vi "Windspeed Warnings.vi"(8 "error in":errorcluster, 11 "Weather Data In":T1={"Current Temperature"=0.0, "Max Temperature"=0.0, "Min Temperature"=0.0, "Temperature Warning?"=FALSE, "Temperature Warning Text"="No Warning", "Current Windspeed"=0.0, "Max Windspeed"=0.0, "Windspeed Warning?"=FALSE, "Windspeed Warning Text"="No Warning"}) -> (0 "error out":errorcluster, 3 "Weather Data Out":T1={"Current Temperature"=0.0, "Max Temperature"=0.0, "Min Temperature"=0.0, "Temperature Warning?"=FALSE, "Temperature Warning Text"="No Warning", "Current Windspeed"=0.0, "Max Windspeed"=0.0, "Windspeed Warning?"=FALSE, "Windspeed Warning Text"="No Warning"})   [LabVIEW 2012]
doc: "This VI is used to determine the string to output to the weather station based on the current wind and limit settings."
uses:
  Weather Data.ctl
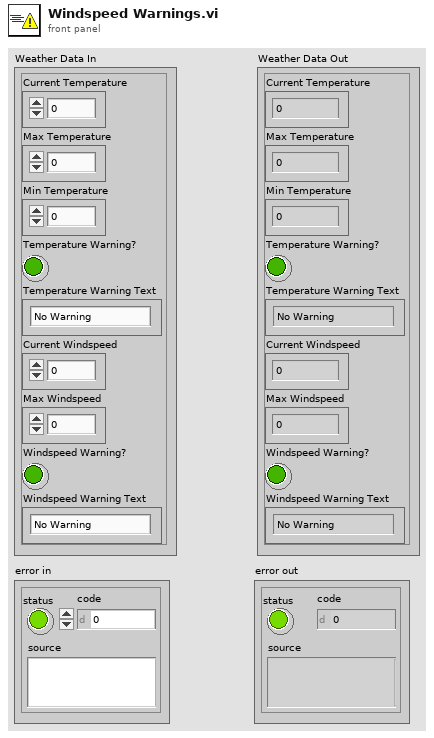
[diagram p1: front panel]
types:
  T1 = typedef "Weather Data.ctl" = cluster{"Current Temperature":dbl, "Max Temperature":dbl, "Min Temperature":dbl, "Temperature Warning?":bool, "Temperature Warning Text":string, "Current Windspeed":dbl, "Max Windspeed":dbl, "Windspeed Warning?":bool, "Windspeed Warning Text":string}
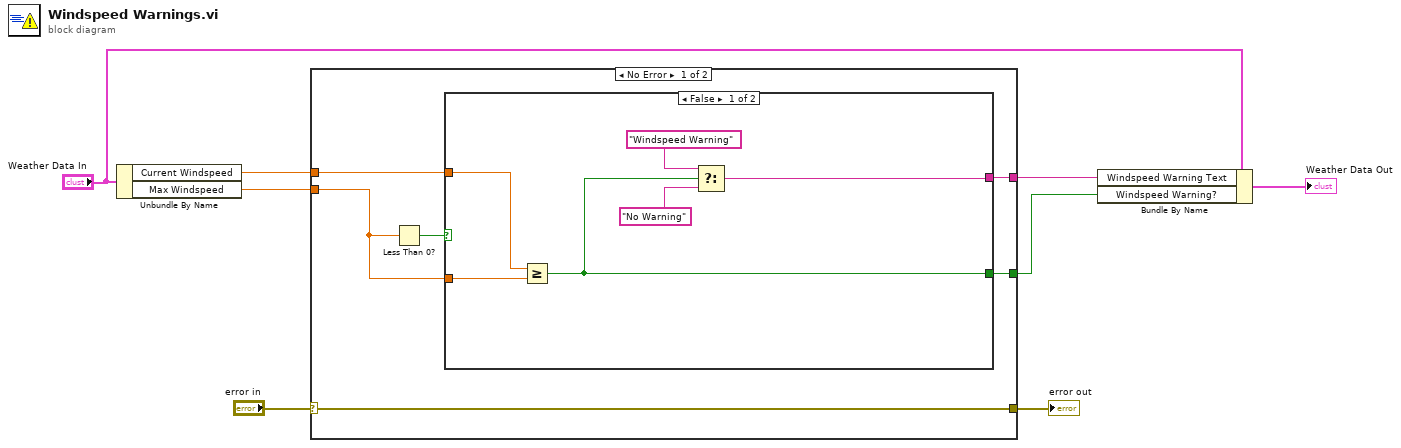
[diagram p0: block diagram]
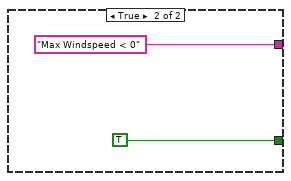
[diagram p2: hidden frame]
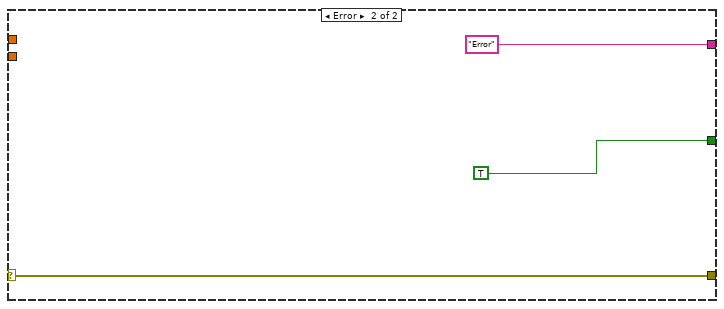
[diagram p3: hidden frame]
diagram:
  n1 = Unbundle By Name("Weather Data In") -> ("Current Windspeed"=w6:dbl, "Max Windspeed"=w5:dbl)
  n2 = case shown="No Error" "error in" {
    selector: "error in" -> [w11 w25]
    tunnel: [w14 "Error" ("f")] -> w3
    tunnel: [w13 TRUE] -> w2
    tunnel: [w11 w25] -> w7
    tunnel: w6 -> [w10 _]
    tunnel: w5 -> [w9 _]
    frame No Error {
      n3 = Less Than 0?(x=w9) -> (x < 0?=w12:bool)
      n4 = case shown="False" w12 {
        tunnel: [w16 "Max Windspeed < 0" ("f")] -> w14
        tunnel: [w15 TRUE] -> w13
        tunnel: w9 -> [w20 _]
        tunnel: w10 -> [w17 _]
        frame False {
          n5 = Greater Or Equal?(x=w17, y=w20) -> (x >= y?=w15:bool)
          n6 = Select(t="Windspeed Warning", s=w15, f="No Warning") -> (s? t:f=w16:string)
        }
        frame True {
        }
      }
    }
    frame Error {
    }
  }
  "error out" <- w7
  n7 = Bundle By Name(cluster="Weather Data In", "Windspeed Warning Text"=w3, "Windspeed Warning?"=w2) -> (→"Weather Data Out":T1)
